vi "ConfigureDlg.vi"(8 "error in (no error)":errorcluster, 11 "StandardFunction in":refnum<class "StandardFunction.lvclass">) -> (0 "error out":errorcluster, 2 "Changed":bool, 3 "StandardFunction out":refnum<class "StandardFunction.lvclass">)   [LabVIEW 2014, in "Functions.lvlib" / "StandardFunction.lvclass"]
uses:
  StandardFunction.lvclass
  TypeDefs/StdWfrms.ctl
  TypeDefs/StdWfrm.ctl
  StandardFunction.lvclass/StandardFunction.ctl
  FunctionBaseClass/FunctionBase.lvclass/FunctionBase.ctl
  FunctionBaseClass/Accessors/Read FunctionIniFilePath.vi
  Accessors/Write StandardWfrms.vi
  Accessors/Read StandardWfrms.vi
  <vilib>/Utility/config.llb/NI_LVConfig.lvlib
panel:
  in  "btnDone":bool
  in  "btnCancel":bool
  in  "StandardWfrms":T1
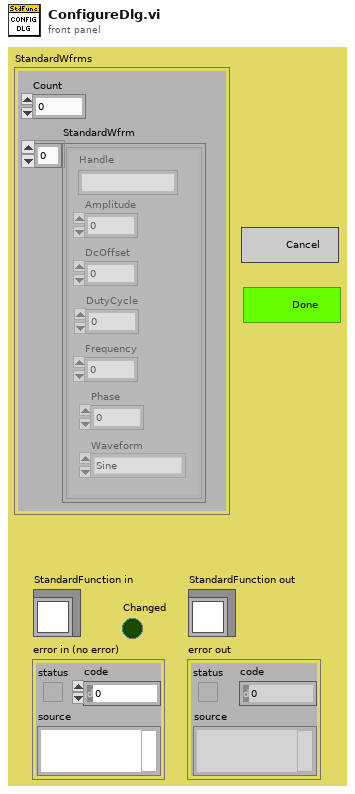
[diagram p1: front panel]
types:
  T1 = typedef "Functions.lvlib/StandardFunction.lvclass/StdWfrms.ctl" = cluster{"Count":u16, "StandardWfrm":T2[]}
  T2 = typedef "Functions.lvlib/StandardFunction.lvclass/StdWfrm.ctl" = cluster{"Amplitude":dbl, "DcOffset":dbl, "DutyCycle":dbl, "Frequency":dbl, "Phase":dbl, "Waveform":enum16{"Sine", "Square", "Triangle", "Ramp Up", "Ramp Down", "DC"}, "Handle":string}
  T3 = typedef "NI_LVConfig.lvlib/Config Data RefNum.ctl" = refnum<k1>
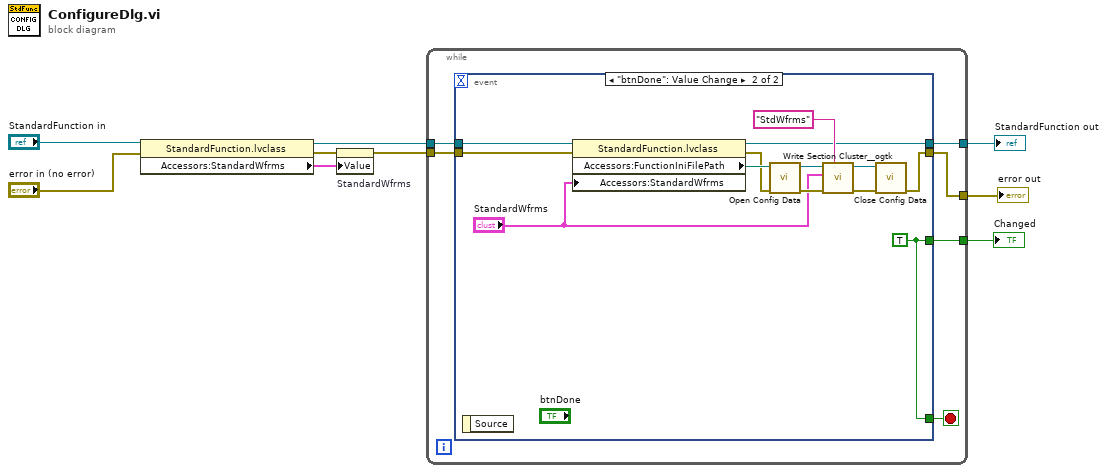
[diagram p0: block diagram]
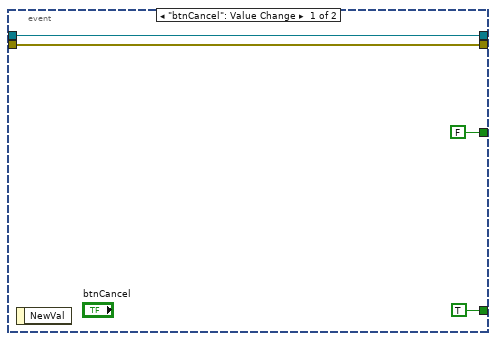
[diagram p2: hidden frame]
diagram:
  n1 = property class="StandardFunction.lvclass"(reference="StandardFunction in", error in="error in (no error)") -> (reference out=w4:refnum<class "StandardFunction.lvclass">, error out=w6:errorcluster, "Accessors:StandardWfrms"=w7:T1)
  n2 = property on="StandardWfrms" class="Clust (strict)"(error in=w6, "Value"=w7) -> (error out=w5:errorcluster)  [unwired: 1 in, 1 out]
  n3 = while {
    tunnel: w5 -> [w15]
    tunnel: w4 -> [w14]
    tunnel: [w13] -> w3
    tunnel: [w11] -> w2
    tunnel: [w10] -> w1
    stop <- w12 stop-if-true
    n4 = event shown="[1] \"btnDone\": Value Change" {
      selector: _ -> [_ _]
      dyn-events: _ -> [_ _]
      timeout: _ -> [_ _]
      tunnel: w15 -> [w18 w31]
      tunnel: w14 -> [w19 w32]
      tunnel: [w19 w20] -> w13
      tunnel: [w18 w22] -> w11
      tunnel: [TRUE w21] -> w12
      tunnel: [FALSE w21] -> w10
      event "btnCancel": Value Change {
        n5 = event-data() -> ()  [unwired: 1 in, 1 out]
      }
      event "btnDone": Value Change {
        w21 = TRUE
        n6 = event-data() -> ()  [unwired: 1 in, 1 out]
        n7 = property class="StandardFunction.lvclass"(reference=w32, error in=w31, "Accessors:StandardWfrms"="StandardWfrms") -> (reference out=w20:refnum<class "StandardFunction.lvclass">, error out=w29:errorcluster, "Accessors:FunctionIniFilePath"=w30:path)
        n8 = call <vilib>:"Open Config Data.vi"("error in (no error)"=w29, "configuration file path"=w30) -> ("error out"=w28:errorcluster, "refnum"=w27:T3)  [unwired: 7 in, 1 out]
        n9 = call <userlib>:"Write Section Cluster__ogtk.vi"("section (optional)"="StdWfrms", "error in (no error)"=w28, "Section Formatted Cluster"="StandardWfrms", "refnum"=w27) -> ("error out"=w24:errorcluster, "dup refnum"=w23:T3)  [unwired: 6 in]
        n10 = call <vilib>:"Close Config Data.vi"("error in (no error)"=w24, "refnum"=w23) -> ("error out"=w22:errorcluster)  [unwired: 8 in, 1 out]
      }
    }
  }
  "error out" <- w2
  "StandardFunction out" <- w3
  "Changed" <- w1
